vi "Make_Benchmark_Results_Dir.vi"(11 "Caller Path":path) -> (2 "Caller FP Image Path":path, 3 "CSV_File":path)   [LabVIEW 2020]
uses:
  <vilib>/Ngene/CuLab - GPU Accelerated Toolkit/Toolkit/CuLab.lvlib
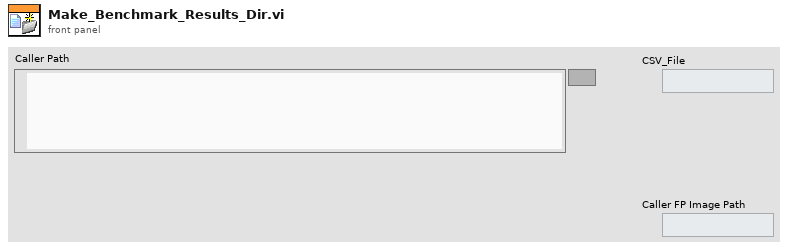
[diagram p1: front panel]
types:
  T1 = typedef "CuLab.lvlib/Properties.ctl" = cluster{"Device ID":i32, "Name":string}
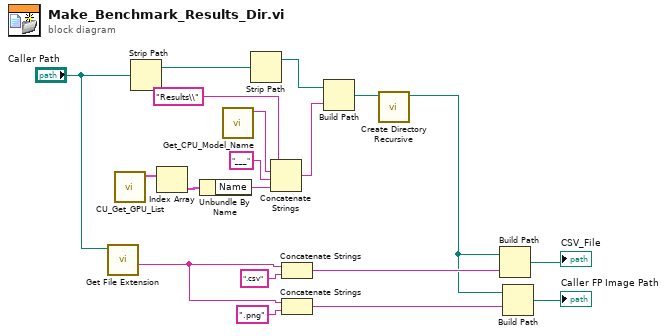
[diagram p0: block diagram]
diagram:
  n1 = call <vilib>:"Get File Extension.vi"("file"="Caller Path") -> ("filename without extension"=w15:string)  [unwired: 6 in, 4 out]
  n2 = call <vilib>:"CU_Get_GPU_List.vi"() -> ("Devices"=w8:T1[])  [unwired: 10 in, 1 out]
  n3 = Strip Path(path="Caller Path") -> (stripped path=w12:path)  [unwired: 1 out]
  n4 = Index Array(array=w8) -> (element=w7:T1)  [unwired: 1 in]
  n5 = Unbundle By Name(w7) -> ("Name"=w4:string)
  n6 = call "Get_CPU_Model_Name.vi"() -> ("CPU Model"=w6:string)  [unwired: 11 in]
  n7 = Strip Path(path=w12) -> (stripped path=w13:path)  [unwired: 1 out]
  n8 = Concatenate Strings("Results\\" ("string"), w6, "___" ("string"), w4) -> (w3:string)
  n9 = Concatenate Strings(w15, ".csv" ("string")) -> (w10:string)
  n10 = Concatenate Strings(w15, ".png" ("string")) -> (w17:string)
  n11 = Build Path(base path=w13, name or relative path=w3) -> (appended path=w16:path)
  n12 = call <vilib>:"Create Directory Recursive.vi"("directory"=w16) -> ("directory copy"=w2:path)  [unwired: 4 in, 2 out]
  n13 = Build Path(base path=w2, name or relative path=w10) -> (appended path=→"CSV_File":path)
  n14 = Build Path(base path=w2, name or relative path=w17) -> (appended path=→"Caller FP Image Path":path)
